vi "Menu_Enable.vi"(7 "Ctrl":string, 8 "error in (no error)":errorcluster, 10 "DB Ref":T1, 11 "String":string) -> (0 "error out":errorcluster)   [LabVIEW 2017, in "tagdb-RefMgr Operations.lvlib"]
uses:
  <userlib>/_NEVSTOP/TagDB/Typedef/TagDB.ctl
  00d0da00-135c-4b50-b029-f1f1f0d03544.vi
  3fef5895-5f1b-4d45-a284-c279625095f7.vi
  4c542a80-f847-4821-836c-1c9f0a826a9d.vi
  00d0da00-135c-4b50-b029-f1f1f0d03544.vi/1b47866c-8e2d-43a7-815f-8cf18635e5a1.vi
  4c542a80-f847-4821-836c-1c9f0a826a9d.vi/1b47866c-8e2d-43a7-815f-8cf18635e5a1.vi
  <userlib>/_NEVSTOP/TagDB/_Support/Error/_Clear Errors.vi
  00d0da00-135c-4b50-b029-f1f1f0d03544.vi/1b47866c-8e2d-43a7-815f-8cf18635e5a1.vi/29b2ea6d-6d7f-4e4a-ad31-a5cb760462c7.vi
  <userlib>/_NEVSTOP/TagDB/API/TagDB-Status.vi
  4c542a80-f847-4821-836c-1c9f0a826a9d.vi/1b47866c-8e2d-43a7-815f-8cf18635e5a1.vi/29b2ea6d-6d7f-4e4a-ad31-a5cb760462c7.vi
  <userlib>/_NEVSTOP/TagDB/_Support/DataAccess/_NameCacher.vi
  <userlib>/_NEVSTOP/TagDB/_Support/Change Detector/TagDB dbChanged.vi
  <userlib>/_NEVSTOP/TagDB/_Support/DataAccess/TagDB Ref to DVR.vi
  <userlib>/_NEVSTOP/TagDB/_Support/Error/_[error50000]Invalid DB REF.vi
  <userlib>/_NEVSTOP/TagDB/_Support/URL/TRIM-BOTH-SPACE.vi
  <userlib>/_NEVSTOP/TagDB/_Support/Error/_[error50002]Invalid DataType.vi
  tagdb-RefMgr Operations.lvlib
  <userlib>/_NEVSTOP/TagDB/TagDB.lvlib
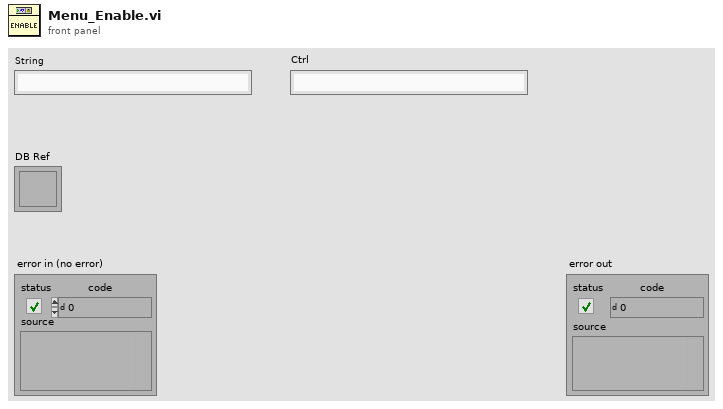
[diagram p1: front panel]
types:
  T1 = typedef "TagDB.lvlib/TagDB.ctl" = refnum<k1>
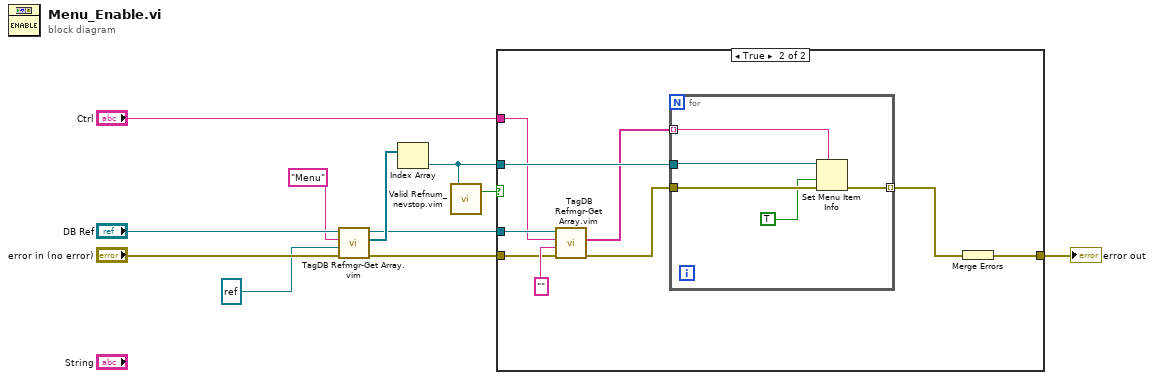
[diagram p0: block diagram]
diagram:
  n1 = call "TagDB Refmgr-Get Array.vim"("error in (no error)"="error in (no error)", "Type"=refnum<k9> refnum ("menu reference"), "RegExp"="Menu", "DB Ref"="DB Ref") -> ("error out"=w2:errorcluster, "References"=w7:refnum<k9>[], "DB Ref(dup)"=w6:T1)  [unwired: 4 in, 1 out]
  n2 = Index Array(array=w7) -> (element=w5:refnum<k9>)  [unwired: 1 in]
  n3 = call "Valid Refnum_nevstop.vim"("number/path/refnum"=w5) -> ("Valid Number/Path/Refnum"=w1:bool)  [unwired: 2 in]
  n4 = case shown="True" w1 {
    tunnel: w6 -> [_ w21]
    tunnel: w5 -> [_ w20]
    tunnel: "Ctrl" -> [_ w18]
    tunnel: [w12 w15] -> w3
    tunnel: w2 -> [w12 w14]
    frame False {
    }
    frame True {
      n5 = call "TagDB Refmgr-Get Array.vim"("error in (no error)"=w14, "Type"="" ("RegExp"), "RegExp"=w18, "DB Ref"=w21) -> ("error out"=w13:errorcluster, "References"=w17:string[])  [unwired: 4 in, 2 out]
      n6 = for {
        tunnel: w20 -> [w26]
        tunnel: w17 -> [w25] mode=indexing
        tunnel: w13 -> [w24]
        tunnel: [w23] -> w16 mode=indexing
        n7 = Set Menu Item Info(7:w25, 8:w24, 9:TRUE ("checked"), 11:w26) -> (0:w23:errorcluster)  [unwired: 3 in, 1 out]
      }
      n8 = Merge Errors(w16) -> (w15:errorcluster)
    }
  }
  "error out" <- w3
